vi "test Write Data To File.vi"(8 "error in (no error)":errorcluster, 11 "TestCase in":refnum<class "WriteFileTests.lvclass">) -> (0 "error out":errorcluster, 3 "TestCase out":refnum<class "WriteFileTests.lvclass">)   [LabVIEW 2014, in "WriteFileTests.lvclass"]
uses:
  WriteFileTests.lvclass
  <vilib>/addons/_JKI Toolkits/VI Tester/TestCase.llb/TestCase.lvclass
  SPLAT/Position.lvclass
panel:
  in  "file path (use dialog)":path=path "D:/SPLAT-tests/Write File Test/WriteFileTests/write_data_to_file_testfile.txt"
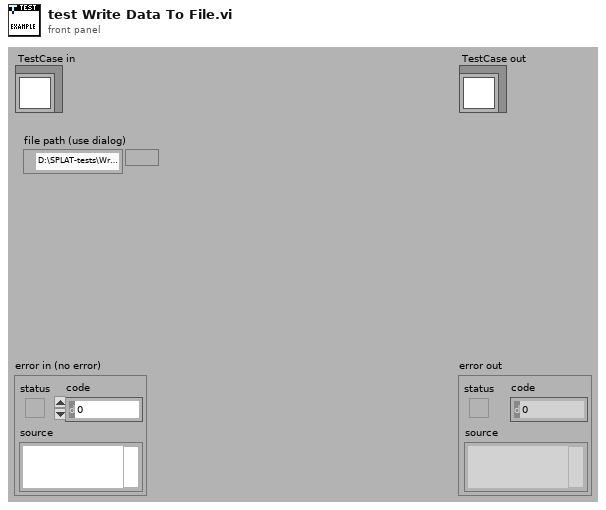
[diagram p1: front panel]
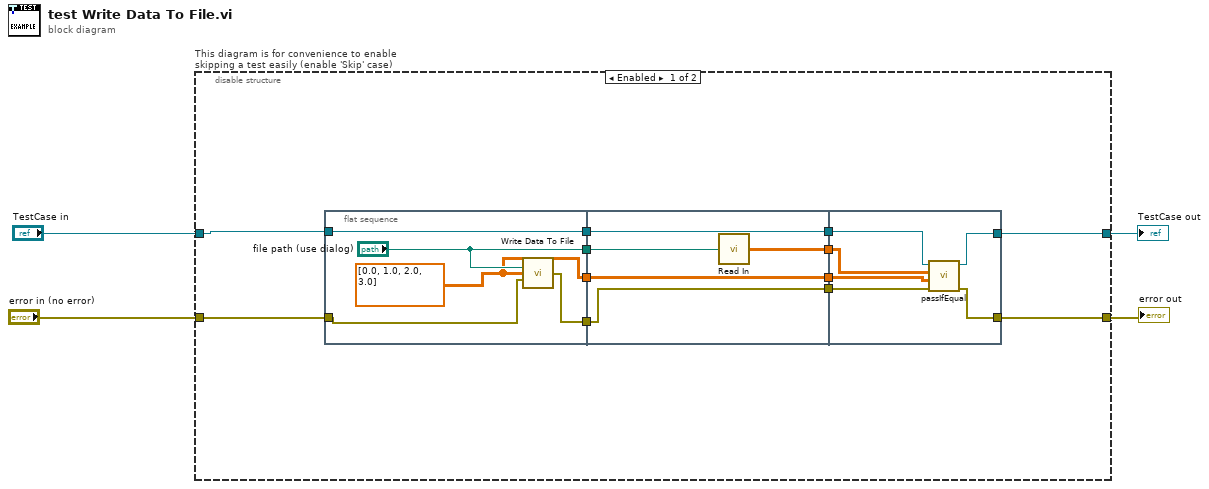
[diagram p0: block diagram]
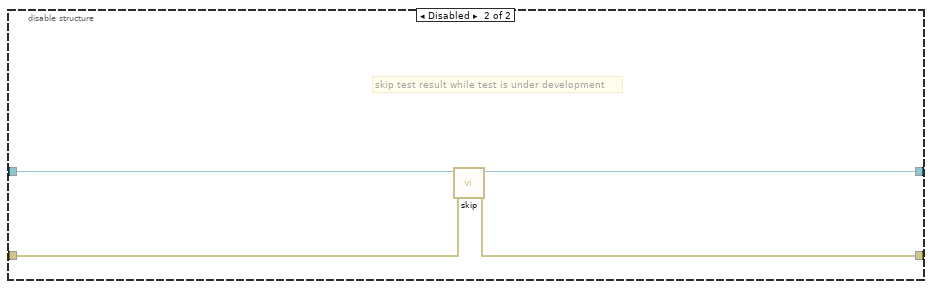
[diagram p2: hidden frame]
diagram:
  n1 = disable-structure "This diagram is for convenience to enable skipping a test easily (enable 'Skip' case)" shown="Enabled" {
    disable-tunnel: "TestCase in" -> [w7 w36]
    disable-tunnel: [w5 w34] -> w1
    disable-tunnel: [w13 w35] -> w3
    disable-tunnel: "error in (no error)" -> [w16 w33]
    frame Enabled {
      n2 = flat-sequence {
        tunnel: w16 -> [w21]
        tunnel: [w20] -> w15
        tunnel: ["file path (use dialog)"] -> w12
        tunnel: [w18] -> w9
        tunnel: w7 -> [w17]
        tunnel: [w17] -> w6
        tunnel: w15 -> [w26]
        tunnel: [w26] -> w14
        tunnel: w12 -> [w25]
        tunnel: [w24] -> w11
        tunnel: [w23] -> w10
        tunnel: w9 -> [w23]
        tunnel: [w22] -> w8
        tunnel: w6 -> [w22]
        tunnel: w14 -> [w32]
        tunnel: [w31] -> w13
        tunnel: w11 -> [w30]
        tunnel: w10 -> [w29]
        tunnel: w8 -> [w28]
        tunnel: [w27] -> w5
        frame #0 {
          w18 = dbl[][] [[0.0, 1.0, 2.0, 3.0]] ("Array")
          n3 = call "Write Data To File.vi"("file path (use dialog)"="file path (use dialog)", "Array"=w18, "error in"=w21) -> ("error out"=w20:errorcluster)  [unwired: 12 in]
        }
        frame #1 {
          n4 = call "Read In.vi"("File path"=w25) -> ("DataOut [tagID, anchorID, distance, time]"=w24:dbl[][])  [unwired: 14 in]
        }
        frame #2 {
          n5 = call-dynamic "passIfEqual.vi"("error in (no error)"=w32, "y"=w29, "x"=w30, "TestCase in"=w28) -> ("error out"=w31:errorcluster, "TestCase out"=w27:refnum<class "WriteFileTests.lvclass">)  [unwired: 6 in]
        }
      }
    }
    frame Disabled {
      # "skip test result while test is under development"
      n6 = call <vilib>:"skip.vi"("error in (no error)"=w33, "TestCase in"=w36) -> ("error out"=w35:errorcluster, "TestCase out"=w34:refnum<class "WriteFileTests.lvclass">)  [unwired: 8 in]
    }
  }
  "error out" <- w3
  "TestCase out" <- w1
